vi "Calc - DeltaB.vi"(11 "PBMeas P":dbl) -> (3 "Delta B":dbl)   [LabVIEW 2018, in "Controller (Host).lvlib"]
uses:
  Controller (Host).lvlib
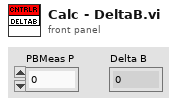
[diagram p1: front panel]
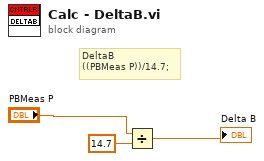
[diagram p0: block diagram]
diagram:
  # "DeltaB\n((PBMeas P))/14.7;"
  n1 = Divide(x="PBMeas P", y=14.7) -> (x/y=→"Delta B":dbl)
